vi "Using Analysis tools (Waveform data type).vi"() -> ()   [LabVIEW 2020]
uses:
  <vilib>/DAQmx/miscellaneous.llb/DAQmx Fill In Error Info.vi
  <vilib>/DAQmx/create/channels.llb/DAQmx Create Channel (AI-Temperature-Thermocouple).vi
  <vilib>/DAQmx/configure/timing.llb/DAQmx Timing (Sample Clock).vi
  <vilib>/DAQmx/read.llb/DAQmx Read (Analog Wfm 1Chan NSamp).vi
  <resource>/objmgr/daqmx.rc
panel:
  out "Acquired Signal":waveform(dbl)(graph)
  in  "Stop":bool
  out "Actual Sample Rate (Hz)":dbl
  in  "Number of Samples":i32=1000
  in  "Desired Sample Rate (Hz)":dbl=1000.0
  in  "Physical Channel":tag="PCI-6221/ai0"
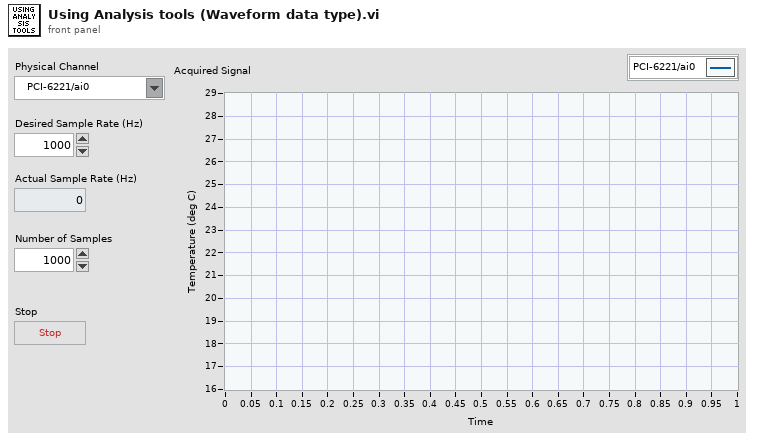
[diagram p1: front panel]
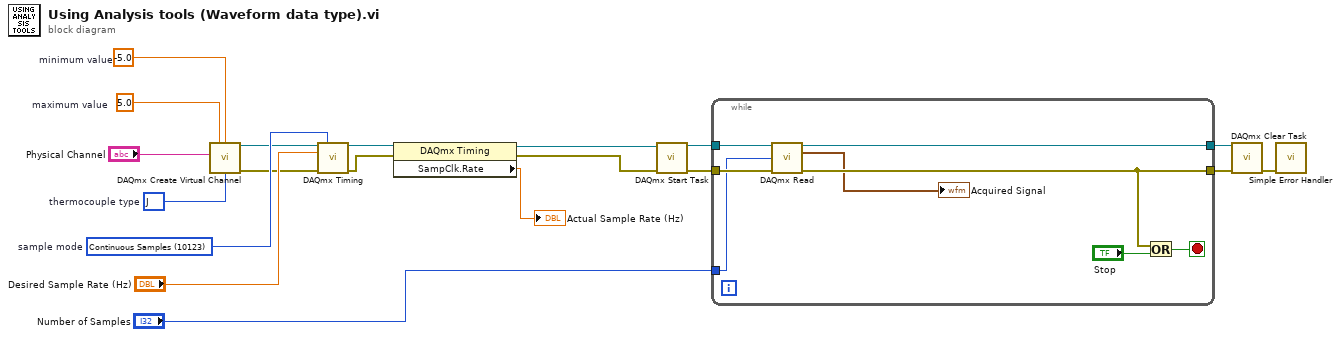
[diagram p0: block diagram]
diagram:
  w1 = 10072 items=["J"=10072, "K"=10073, "N"=10077, "R"=10082, "S"=10085, "T"=10086, "B"=10047, "E"=10055]  # thermocouple type
  w16 = 10123 items=["Finite Samples"=10178, "Continuous Samples"=10123, "Hardware Timed Single Point"=12522]  # sample mode
  w18 = 5.0  # maximum value
  w19 = -5.0  # minimum value
  n1 = call-poly <vilib>:"DAQmx Create Virtual Channel.vi"("maximum value"=w18, "minimum value"=w19, "physical channels"="Physical Channel", "thermocouple type"=w1) -> ("task out"=w14:refnum<k21>, "error out"=w13:errorcluster)  [unwired: 10 in]
  n2 = call-poly <vilib>:"DAQmx Timing.vi"("task/channels in"=w14, "sample mode"=w16, "rate"="Desired Sample Rate (Hz)", "error in"=w13) -> ("task out"=w12:refnum<k21>, "error out"=w11:errorcluster)  [unwired: 10 in]
  n3 = property class="DAQmx Timing"(reference=w12, error in=w11) -> (reference out=w9:refnum<k21>, error out=w8:errorcluster, "SampClk.Rate"=→"Actual Sample Rate (Hz)":dbl)
  n4 = call <vilib>:"DAQmx Start Task.vi"("task/channels in"=w9, "error in"=w8) -> ("task out"=w7:refnum<k21>, "error out"=w6:errorcluster)  [unwired: 12 in]
  n5 = while {
    tunnel: w7 -> [w27]
    tunnel: w6 -> [w26]
    tunnel: "Number of Samples" -> [w25]
    tunnel: [w24] -> w4
    tunnel: [w23] -> w3
    stop <- w21 stop-if-true
    n6 = call-poly <vilib>:"DAQmx Read.vi"("task/channels in"=w27, "number of samples per channel"=w25, "error in"=w26) -> ("task out"=w24:refnum<k21>, "data"=→"Acquired Signal":waveform(dbl), "error out"=w23:errorcluster)  [unwired: 10 in]
    n7 = Or(x=w23, y="Stop") -> (x .or. y?=w21:bool)
  }
  n8 = call <vilib>:"DAQmx Clear Task.vi"("task in"=w4, "error in"=w3) -> ("error out"=w2:errorcluster)  [unwired: 13 in]
  n9 = call <vilib>:"Simple Error Handler.vi"("error in (no error)"=w2) -> ()  [unwired: 4 in, 5 out]
